vi "Test_Connect_Connector_Pane.vi"   [LabVIEW 2025]
uses:
  8cebb4ce-4f0f-4319-9f7e-82e401bee674.vi
  0e244da9-745b-4f2d-a97c-0de3ccfbb071.vi
  57ba1f44-eecb-4af5-975d-0cda700306c1.vi
  Scripting Server.lvlib
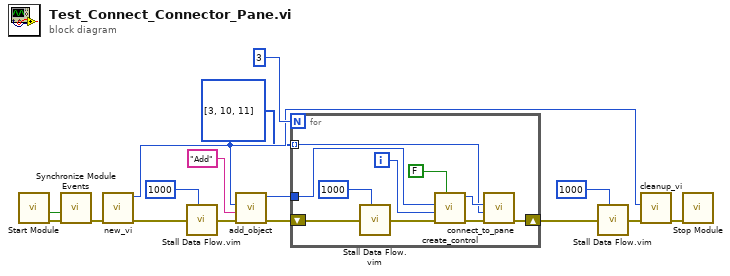
[diagram p0: block diagram]
diagram:
  n1 = call "Start Module.vi"() -> ("error out"=w15:errorcluster, "Wait for Event Sync?"=w16:bool)  [unwired: 7 in, 3 out]
  n2 = call "Synchronize Module Events.vi"("error in"=w15, "Wait for Event Sync?"=w16) -> ("error out"=w14:errorcluster)  [unwired: 9 in]
  n3 = call "new_vi.vi"("error in"=w14) -> ("error out"=w13:errorcluster, "vi_id"=w5:i32)  [unwired: 7 in, 2 out]
  n4 = call "Stall Data Flow.vim"("value in"=w13, "milliseconds to wait"=u32 1000) -> ("value out"=w12:errorcluster)  [unwired: 1 out]
  n5 = call "add_object.vi"("error in"=w12, "object_name"="Add", "diagram_id"=w5) -> ("error out"=w10:errorcluster, "object_id"=w9:i32)  [unwired: 5 in, 2 out]
  n6 = for {
    N: 3 -> [_]
    tunnel: w9 -> [w25]
    shift-right: [w20] -> w6
    shift-left: w10 -> [w26]
    tunnel: i32[] [3, 10, 11] -> [w17] mode=indexing
    i -> [w18]
    n7 = call "Stall Data Flow.vim"("value in"=w26, "milliseconds to wait"=u32 1000) -> ("value out"=w24:errorcluster)  [unwired: 1 out]
    n8 = call "create_control.vi"("constant"=FALSE, "error in"=w24, "terminal_index"=w18, "object_id"=w25) -> ("error out"=w22:errorcluster, "created_object_id"=w19:i32)  [unwired: 5 in, 1 out]
    n9 = call "connect_to_pane.vi"("error in"=w22, "connector_pane_index"=w17, "control_id"=w19) -> ("error out"=w20:errorcluster)  [unwired: 7 in, 1 out]
  }
  n10 = call "Stall Data Flow.vim"("value in"=w6, "milliseconds to wait"=u32 1000) -> ("value out"=w4:errorcluster)  [unwired: 1 out]
  n11 = call "cleanup_vi.vi"("error in"=w4, "vi_reference"=w5) -> ("error out"=w2:errorcluster)  [unwired: 7 in, 2 out]
  n12 = call "Stop Module.vi"("error in"=w2) -> ()  [unwired: 10 in, 1 out]
